vi "ips120 set field sweep rate.vi"(2 "error in (no error)":errorcluster, 3 "field sweep rate (T/min)":dbl, 4 "VISA resource name":refnum<visa-resource-name>) -> (0 "error out":errorcluster, 1 "VISA resource name 2":refnum<visa-resource-name>)   [LabVIEW 2013]
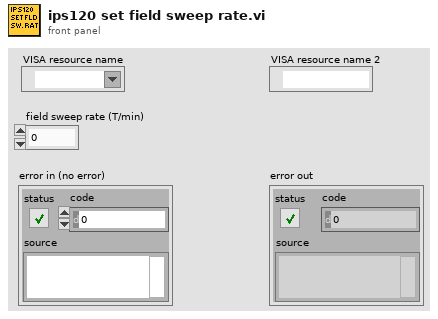
[diagram p1: front panel]
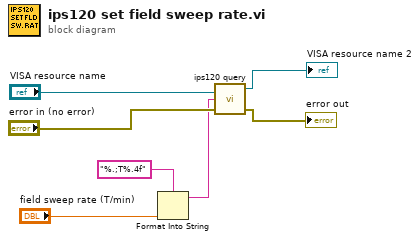
[diagram p0: block diagram]
diagram:
  n1 = Format Into String(format string="%.;T%.4f", "field sweep rate (T/min)") -> (resulting string=w3:string)  [unwired: 2 in, 1 out]
  n2 = call "ips120 query.vi"("error in (no error)"="error in (no error)", "query"=w3, "VISA resource name"="VISA resource name") -> ("error out"=→"error out":errorcluster, "VISA resource name"=→"VISA resource name 2":refnum<visa-resource-name>)  [unwired: 1 out]
